vi "home_channel.vi"(4 "Channel":i32, 6 "file index":i32, 8 "Device ID":refnum<vi>, 9 "Serial #":refnum<vi>, 10 "DAQ channel":tag) -> (1 "Sensor Sampling":waveform(dbl)[](graph), 2 "Zero":i32)   [LabVIEW 2020]
uses:
  <vilib>/Analysis/NI_AALBase.lvlib
  C:/Users/359167/Documents/LabVIEW_ws/Thorlabs.MotionControl.KCube.InertialMotorCLI.dll
  359167/Documents/LabVIEW_ws/Thorlabs.MotionControl.KCube.InertialMotorCLI.dll
  <vilib>/DAQmx/read.llb/DAQmx Read (Analog 1D Wfm NChan NSamp).vi
  <vilib>/DAQmx/create/channels.llb/DAQmx Create Channel (AI-Voltage-Basic).vi
  <vilib>/DAQmx/configure/timing.llb/DAQmx Timing (Sample Clock).vi
  <vilib>/Utility/file.llb/Read Delimited Spreadsheet (DBL).vi
  <vilib>/Analysis/baseanly.llb/Mean (DBL).vi
panel:
  in  "Path":path=path "C:/Users/359167/Documents/saved_position.csv"
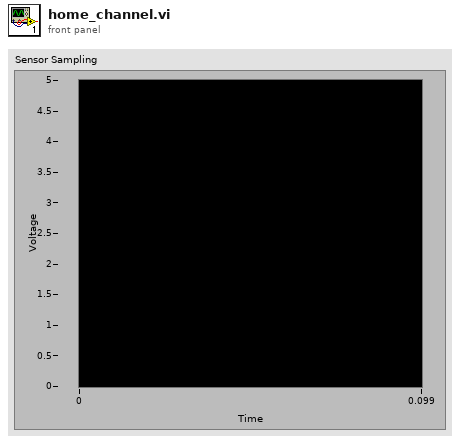
[diagram p1: front panel]
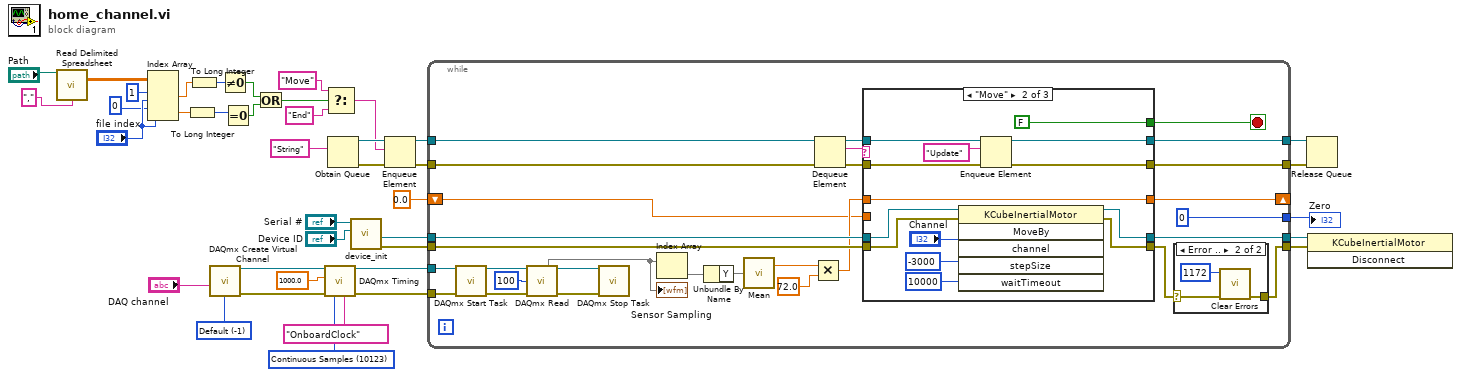
[diagram p0: block diagram]
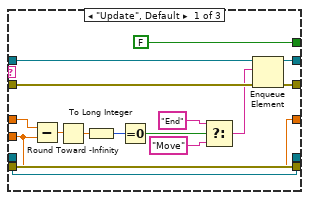
[diagram p3: hidden frame]
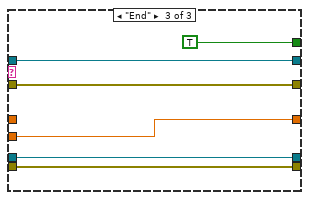
[diagram p4: hidden frame]
diagram:
  w32 = -1 items=["Default"=-1, "RSE"=10083, "NRSE"=10078, "Differential"=10106, "Pseudodifferential"=12529] ("input terminal configuration")
  w33 = 10123 items=["Finite Samples"=10178, "Continuous Samples"=10123, "Hardware Timed Single Point"=12522] ("sample mode")
  n1 = call-poly <vilib>:"Read Delimited Spreadsheet.vi"("file path (dialog if empty)"="Path", "delimiter (\\t)"="," ("delimiter (\\t)")) -> ("all rows"=w21:dbl[][])  [unwired: 8 in, 5 out]
  n2 = Index Array(array=w21, index (row) #1=1 ("channel"), index (col) #1="file index", index (row) #2=0 ("disabled index (col)"), index (col) #2="file index") -> (element #1=w19:dbl, element #2=w15:dbl)
  n3 = To Long Integer(number=w15) -> (32bit integer=w14:i32)
  n4 = To Long Integer(number=w19) -> (32bit integer=w20:i32)
  n5 = call-poly <vilib>:"DAQmx Create Virtual Channel.vi"("input terminal configuration"=w32, "physical channels"="DAQ channel") -> ("task out"=w28:refnum<k21>, "error out"=w29:errorcluster)  [unwired: 12 in]
  n6 = Not Equal To 0?(x=w20) -> (x != 0?=w13:bool)
  n7 = Equal To 0?(x=w14) -> (x = 0?=w12:bool)
  n8 = Or(x=w13, y=w12) -> (x .or. y?=w11:bool)
  n9 = call-poly <vilib>:"DAQmx Timing.vi"("task/channels in"=w28, "sample mode"=w33, "rate"=1000.0 ("sample rate"), "source"=tag "OnboardClock", "error in"=w29) -> ("task out"=w26:refnum<k21>, "error out"=w25:errorcluster)  [unwired: 9 in]
  n10 = Select(t="Move" ("element"), s=w11, f="End" ("t")) -> (s? t:f=w16:string)
  n11 = Obtain Queue(element data type="String") -> (queue out=w37:refnum<queue>, error out=w36:errorcluster)  [unwired: 4 in, 1 out]
  n12 = call "device_init.vi"("Device ID"="Device ID", "Serial #"="Serial #") -> ("error out"=w4:errorcluster, ".NET Refnum out"=w5:refnum<k24>)  [unwired: 8 in]
  n13 = Enqueue Element(queue=w37, element=w16, error in (no error)=w36) -> (queue out=w35:refnum<queue>, error out=w34:errorcluster)  [unwired: 1 in, 1 out]
  n14 = while {
    shift-right: [w42] -> _
    tunnel: w34 -> [w51]
    tunnel: [w61] -> w39
    tunnel: [w53] -> w38
    tunnel: w35 -> [w52]
    shift-left: 0.0 -> [w41]
    tunnel: [0] -> w24
    tunnel: w26 -> [w65]
    tunnel: w25 -> [w64]
    tunnel: w4 -> [w62]
    tunnel: [w46] -> w6
    tunnel: w5 -> [w63]
    tunnel: [w45] -> w7
    stop <- w67 stop-if-true
    # "Consumer"
    n15 = call <vilib>:"DAQmx Start Task.vi"("task/channels in"=w65, "error in"=w64) -> ("task out"=w57:refnum<k21>, "error out"=w58:errorcluster)  [unwired: 12 in]
    n16 = call-poly <vilib>:"DAQmx Read.vi"("task/channels in"=w57, "number of samples per channel"=100 ("n samples/channel"), "error in"=w58) -> (3:w50, "task out"=w59:refnum<k21>, "error out"=w60:errorcluster)  [unwired: 9 in, 1 out]
    "Sensor Sampling" <- w50
    n17 = call <vilib>:"DAQmx Stop Task.vi"("task/channels in"=w59, "error in"=w60) -> ()  [unwired: 12 in, 2 out]
    n18 = Index Array(array=w50) -> (element=w55)  [unwired: 1 in]
    n19 = Unbundle By Name(w55) -> ("Y"=w54)
    n20 = call-poly <vilib>:"Mean.vi"("X"=w54) -> ("mean"=w43:dbl)  [unwired: 1 out]
    n21 = Multiply(x=w43, y=72.0) -> (x*y=w44:dbl)
    n22 = Dequeue Element(queue=w52, error in (no error)=w51) -> (queue out=w69:refnum<queue>, element=w68:string, error out=w66:errorcluster)  [unwired: 1 in, 1 out]
    n23 = case shown="\"Move\"" w68 {
      tunnel: w69 -> [w87 w101 w105]
      tunnel: [w89 w99 w106] -> w61
      tunnel: [FALSE FALSE TRUE] -> w67
      tunnel: w66 -> [w88 w100 w106]
      tunnel: w62 -> [w85 w92 w108]
      tunnel: [w86 w103 w107] -> w45
      tunnel: [w85 w91 w108] -> w47
      tunnel: w63 -> [w86 w102 w107]
      tunnel: [w84 w98 w105] -> w53
      tunnel: w44 -> [w75 w90 _]
      tunnel: [w74 w90 w104] -> w42
      tunnel: w41 -> [w74 _ w104]
      frame "Update", Default {
        n24 = Subtract(x=w75, y=w74) -> (x-y=w76:dbl)
        n25 = Round Toward -Infinity(1:w76) -> (0:w79:dbl)
        n26 = To Long Integer(number=w79) -> (32bit integer=w78:i32)
        n27 = Equal To 0?(x=w78) -> (x = 0?=w83:bool)
        n28 = Select(t="End", s=w83, f="Move" ("element")) -> (s? t:f=w80:string)
        n29 = Enqueue Element(queue=w87, element=w80, error in (no error)=w88) -> (queue out=w84:refnum<queue>, error out=w89:errorcluster)  [unwired: 1 in, 1 out]
      }
      frame "Move" {
        n30 = invoke class="KCubeInertialMotor" method="MoveBy"(reference=w102, error in=w92, "channel"="Channel", "stepSize"=-3000, "waitTimeout"=10000) -> (reference out=w103:refnum<k24>, error out=w91:errorcluster)  [unwired: 1 in, 4 out]
        n31 = Enqueue Element(queue=w101, element="Update", error in (no error)=w100) -> (queue out=w98:refnum<queue>, error out=w99:errorcluster)  [unwired: 1 in, 1 out]
      }
      frame "End" {
      }
    }
    n32 = case shown="Error .." w47 {
      selector: w47 -> [w70 w72]
      tunnel: [w70 w71] -> w46
      frame No Error {
      }
      frame Error {
        n33 = call <vilib>:"Clear Errors.vi"("error in (no error)"=w72, "specific error code to clear (0: all)"=1172) -> ("error out"=w71:errorcluster)  [unwired: 4 in, 1 out]
      }
    }
  }
  "Zero" <- w24
  n34 = Release Queue(queue=w38, error in (no error)=w39) -> ()  [unwired: 1 in, 3 out]
  n35 = invoke class="KCubeInertialMotor" method="Disconnect"(reference=w7, error in=w6) -> ()  [unwired: 1 in, 3 out]
